vi "MCL Trigger Load Wave Form N.vi"(10 "handle":i32, 11 "axis":u32) -> (3 "function return":i32)   [LabVIEW 2017, in "Madlib.lvlib"]
doc: "MADLIB_API int MCL_Trigger_LoadWaveFormN(unsigned int axis, int handle);"
uses:
  Madlib.lvlib
  Madlib.dll
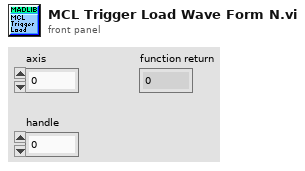
[diagram p1: front panel]
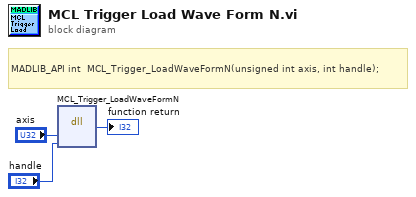
[diagram p0: block diagram]
diagram:
  # "MADLIB_API\tint\t\tMCL_Trigger_LoadWaveFormN(unsigned int axis, int handle);"
  n1 = dll-call lib="C:/Users/francesco/dev/pump-probe/Piezo/lvlib/Madlib.*" fn="MCL_Trigger_LoadWaveFormN"("axis"="axis", "handle"="handle") -> (→"function return":i32)  [unwired: 5 in, 2 out]
